vi "GetSET GRBL last status.vi"(0 "Status in":T1=enum."Alarm", 5 "Current position in":cluster{"X":sgl, "Y":sgl, "Z":sgl}, 7 "Limit switch in":cluster{"X":bool, "Y":bool, "Z":bool}, 9 "Get/Set":enum16{"Get", "Set"}(ring)=enum."Set", 11 "error in (no error)":errorcluster) -> (4 "Status out":T1=enum."Alarm", 6 "Current position out":cluster{"X":sgl, "Y":sgl, "Z":sgl}, 8 "Limit switch out":cluster{"X":bool, "Y":bool, "Z":bool}, 15 "error out":errorcluster)   [LabVIEW 2024, in "GRBL 1.1.lvlib"]
doc: "This VI is use to get the latest status from GRBL.\nThe set is done trough the GET Status.vi.\nThis is usefull when using a different process in parralel and querry what is the status without interfacing the hardware."
uses:
  GRBL 1.1.lvlib
  Status.ctl
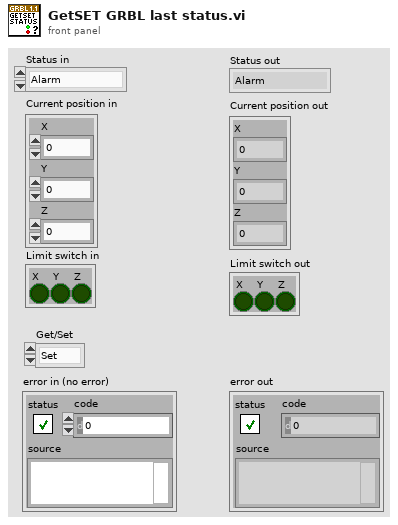
[diagram p1: front panel]
types:
  T1 = typedef "GRBL 1.1.lvlib/Status.ctl" = enum16{"", "Alarm", "Idle", "Run", "Home"}
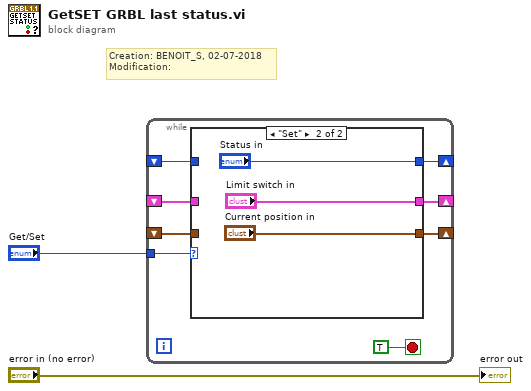
[diagram p0: block diagram]
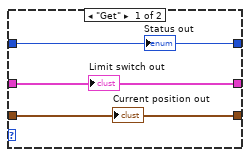
[diagram p2: hidden frame]
diagram:
  # "Creation: BENOIT_S, 02-07-2018\nModification:"
  n1 = while {
    tunnel: "Get/Set" -> [w9]
    shift-right: [w8] -> _
    shift-left: _ -> [w7]
    shift-right: [w5] -> _
    shift-left: _ -> [w4]
    shift-right: [w6] -> _
    shift-left: _ -> [w3]
    stop <- TRUE stop-if-true
    n2 = case shown="\"Set\"" w9 {
      tunnel: [w12 "Current position in"] -> w8
      tunnel: w7 -> [w12 _]
      tunnel: [w13 "Status in"] -> w6
      tunnel: [w11 "Limit switch in"] -> w5
      tunnel: w4 -> [w11 _]
      tunnel: w3 -> [w13 _]
      frame "Get" {
        "Status out" <- w13
        "Current position out" <- w12
        "Limit switch out" <- w11
      }
      frame "Set" {
      }
    }
  }
  "error out" <- "error in (no error)"
